vi "ILABW_SetBounds.vi"(3 "left":i16, 4 "right":i16, 5 "bottom":i16, 6 "top":i16, 7 "viname":string) -> ()   [LabVIEW 2012]
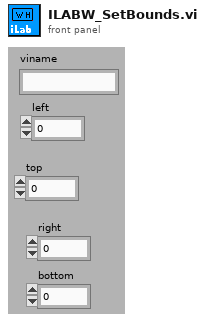
[diagram p1: front panel]
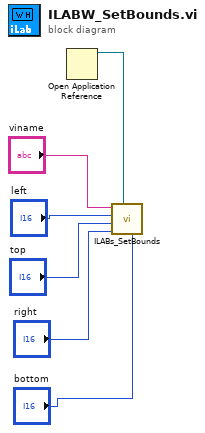
[diagram p0: block diagram]
diagram:
  n1 = Open Application Reference() -> (3:w6:refnum<vi>)  [unwired: 1 in, 4 out]
  n2 = call "ILABs_SetBounds.vi"("viname"="viname", "left"="left", "top"="top", "right"="right", "appRef"=w6, "bottom"="bottom") -> ()  [unwired: 1 out]
